vi "PopOpDebug.vi"(8 "Error In":errorcluster, 11 "Debug in":refnum<class "Debug.lvclass">) -> (0 "Error Out":errorcluster, 3 "Debug out":refnum<class "Debug.lvclass">)   [LabVIEW 2021, in "Debug.lvclass"]
doc: "Debug pop-op with class name."
uses:
  Debug.lvclass
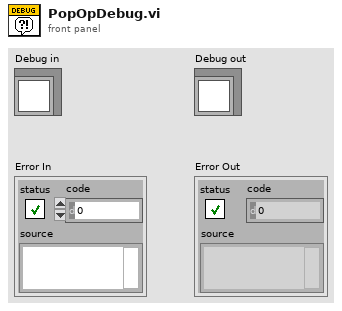
[diagram p1: front panel]
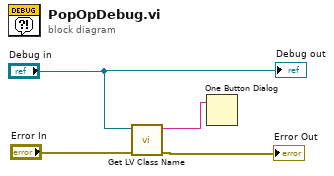
[diagram p0: block diagram]
diagram:
  n1 = call <vilib>:"Get LV Class Name.vi"("error in (no error)"="Error In", "object"="Debug in") -> ("error out"=→"Error Out":errorcluster, "class name"=w1:string)  [unwired: 8 in]
  n2 = One Button Dialog(message=w1) -> ()  [unwired: 1 in, 1 out]
  "Debug out" <- "Debug in"
